vi "LEP_RV_BuildSpec_InitTempValues.vi"(3 "error in (no error)":errorcluster, 4 "Default Values":refnum<vi>[](array[refnum])=[refnum, refnum, refnum, refnum, refnum, refnum, refnum, refnum, refnum, refnum, refnum, refnum, refnum, refnum], 5 "Attribute Name":string[](array[string])) -> (0 "error out":errorcluster, 2 "Attribute Name":string[](array[string]))   [LabVIEW 2011]
uses:
  <vilib>/Platform/EmbProject/Plugins/utilities/LEP_Utilities_GetSetProjectData_Variant.vi
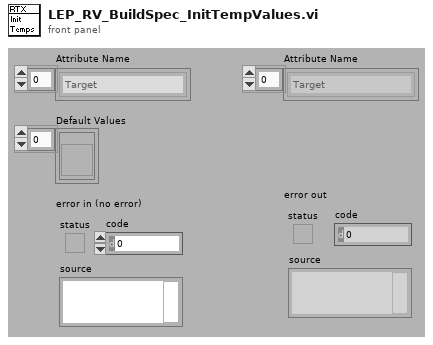
[diagram p1: front panel]
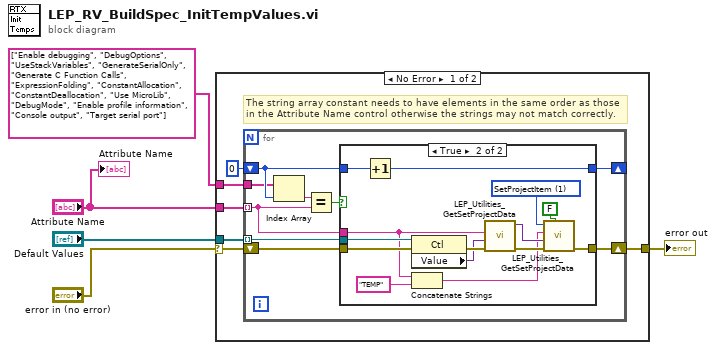
[diagram p0: block diagram]
diagram:
  n1 = case shown="No Error" "error in (no error)" {
    selector: "error in (no error)" -> [w7 w37]
    tunnel: [w11 w37] -> w5
    tunnel: "Attribute Name" -> [w10 _]
    tunnel: "Default Values" -> [w9 _]
    tunnel: string[] ["Enable debugging", "DebugOptions", "UseStackVariables", "GenerateSerialOnly", "Generate C Function Calls", "ExpressionFolding", "ConstantAllocation", "ConstantDeallocation", "Use MicroLib", "DebugMode", "Enable profile information", "Console output", "Target serial port"] -> [w8 _]
    frame No Error {
      # "The string array constant needs to have elements in the same order as those in the Attribute Name control otherwise the strings may not match correctly."
      n2 = for {
        tunnel: w10 -> [w18] mode=indexing
        tunnel: w9 -> [w17] mode=indexing
        tunnel: w8 -> [w13]
        shift-right: [w19] -> w11
        shift-left: w7 -> [w20]
        shift-right: [w15] -> _
        shift-left: 0 -> [w14]
        n3 = Index Array(array=w13, index=w14) -> (element=w12:string)
        n4 = Equal?(x=w12, y=w18) -> (x = y?=w16:bool)
        n5 = case shown="True" w16 {
          tunnel: w20 -> [w22 w36]
          tunnel: w17 -> [_ w34]
          tunnel: [w22 w27] -> w19
          tunnel: w18 -> [_ w26]
          tunnel: w14 -> [w21 w25]
          tunnel: [w21 w24] -> w15
          frame False {
          }
          frame True {
            w32 = u16 1 items=["GetProjectItem", "SetProjectItem"] ("Command")
            n6 = Increment(x=w25) -> (x+1=w24:i32)
            n7 = property class="Ctl"(reference=w34, error in=w36) -> (error out=w35:errorcluster, "Value"=w33:variant)  [unwired: 1 out]
            n8 = Concatenate Strings(w26, "TEMP" ("string")) -> (w28:string)
            n9 = call-poly <vilib>:"LEP_Utilities_GetSetProjectData.vi"("error in"=w35, "Variant In"=w33, "ItemName"=w26) -> ("error out"=w31:errorcluster, "Variant Out"=w30:variant)  [unwired: 2 in, 5 out]
            n10 = call-poly <vilib>:"LEP_Utilities_GetSetProjectData.vi"("Is Persistent"=FALSE, "error in"=w31, "Variant In"=w30, "ItemName"=w28, "Command"=w32) -> ("error out"=w27:errorcluster)  [unwired: 1 in, 5 out]
          }
        }
      }
    }
    frame Error {
    }
  }
  "error out" <- w5
  "Attribute Name" <- "Attribute Name"
